vi "imageTrace.vi"() -> ()   [LabVIEW 2012]
uses:
  <vilib>/vision/NI_Vision_Development_Module.lvlib
panel:
  in  "Stop (F)":bool
  out "Image Out":T1(plugin-control)
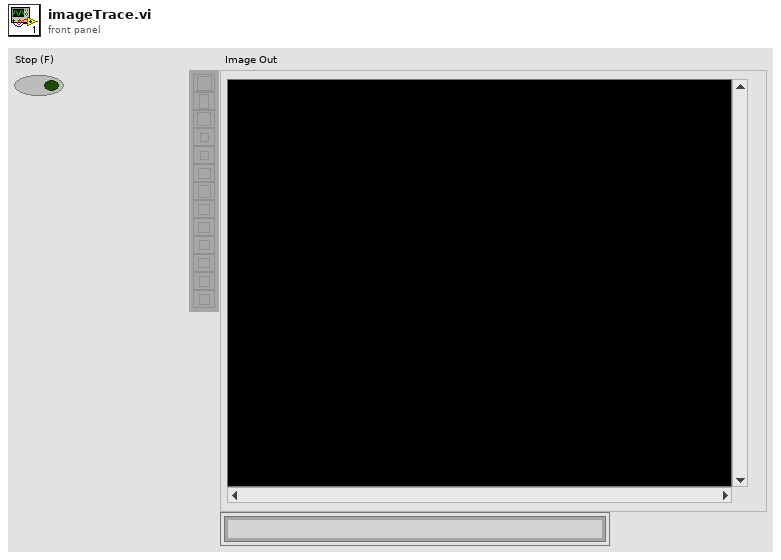
[diagram p1: front panel]
types:
  T1 = typedef "IMAQ Image.ctl" = refnum<image>
  T2 = typedef "Image Type" = u32
  T3 = cluster{"Position":cluster{"x":sgl, "y":sgl}, "Angle":sgl, "Scale":sgl, "Score":sgl, "Bounding Box":cluster{"x":sgl, "y":sgl}[]}[]
  T4 = cluster{"Matches (Pattern Matching 1)[0]":cluster{"Position":cluster{"x":sgl, "y":sgl}, "Angle":sgl, "Scale":sgl, "Score":sgl, "Bounding Box":cluster{"x":sgl, "y":sgl}[]}, "Matches (Pattern Matching 1)[1]":cluster{"Position":cluster{"x":sgl, "y":sgl}, "Angle":sgl, "Scale":sgl, "Score":sgl, "Bounding Box":cluster{"x":sgl, "y":sgl}[]}, "Matches (Pattern Matching 1)[2]":cluster{"Position":cluster{"x":sgl, "y":sgl}, "Angle":sgl, "Scale":sgl, "Score":sgl, "Bounding Box":cluster{"x":sgl, "y":sgl}[]}, "Matches (Pattern Matching 1)[3]":cluster{"Position":cluster{"x":sgl, "y":sgl}, "Angle":sgl, "Scale":sgl, "Score":sgl, "Bounding Box":cluster{"x":sgl, "y":sgl}[]}}
  T5 = cluster{"Bounding Box[0]":cluster{"x":sgl, "y":sgl}, "Bounding Box[1]":cluster{"x":sgl, "y":sgl}, "Bounding Box[2]":cluster{"x":sgl, "y":sgl}, "Bounding Box[3]":cluster{"x":sgl, "y":sgl}, "Bounding Box[4]":cluster{"x":sgl, "y":sgl}, "Bounding Box[5]":cluster{"x":sgl, "y":sgl}, "Bounding Box[6]":cluster{"x":sgl, "y":sgl}, "Bounding Box[7]":cluster{"x":sgl, "y":sgl}, "Bounding Box[8]":cluster{"x":sgl, "y":sgl}}
  T6 = cluster{"[0]":sgl, "[1]":sgl, "[2]":sgl, "[3]":sgl}
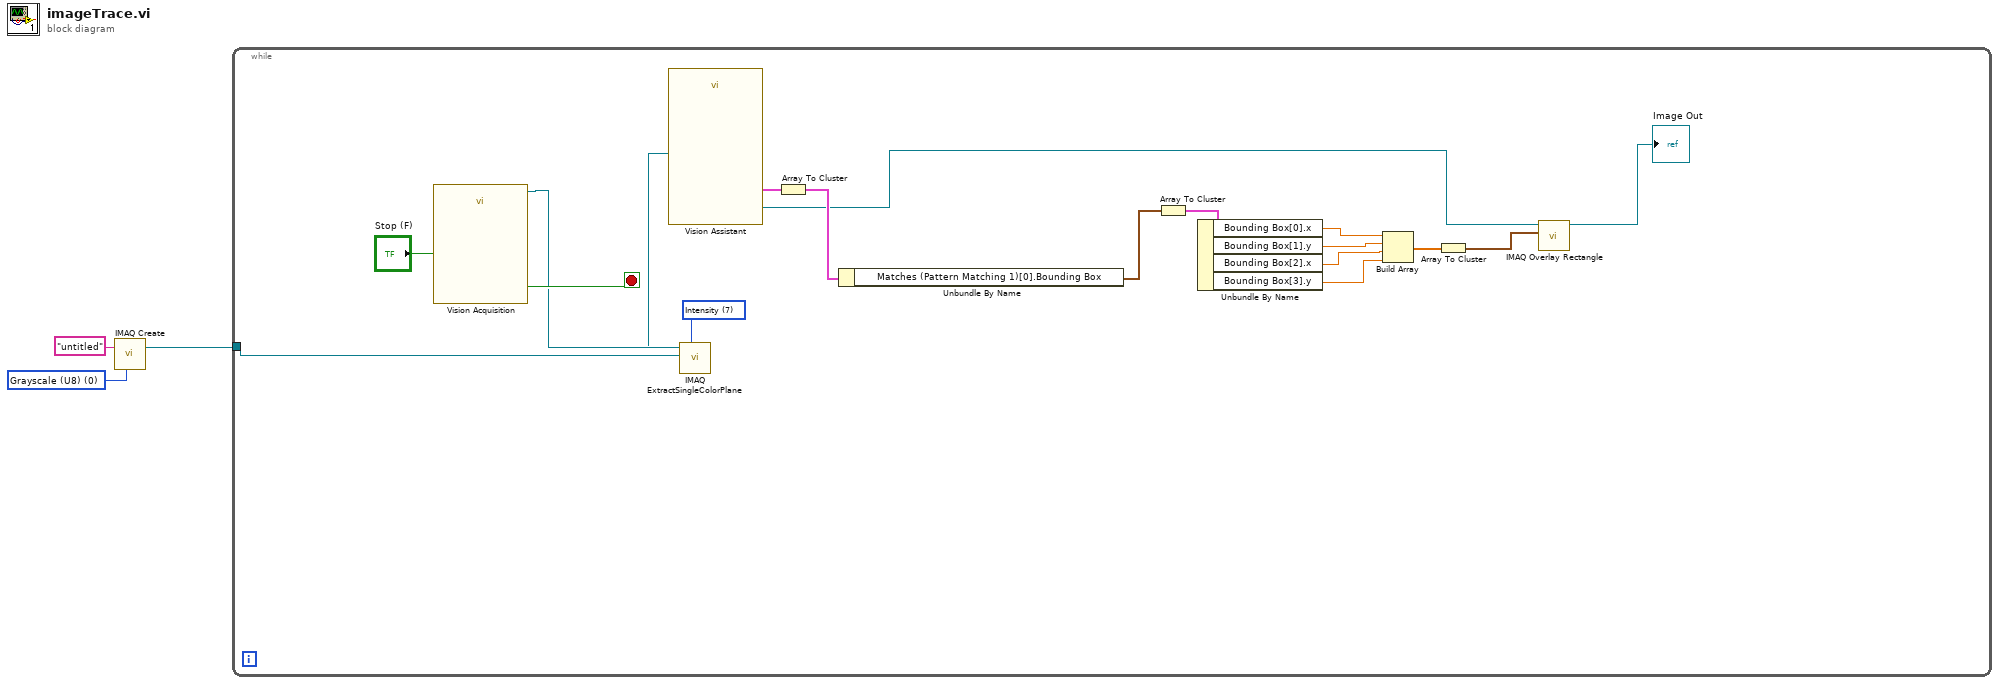
[diagram p0: block diagram]
diagram:
  w2 = T2 0 items=["Grayscale (U8)", "Grayscale (I16)", "Grayscale (SGL)", "Complex (CSG)", "RGB (U32)", "HSL (U32)", "RGB (U64)", "Grayscale (U16)"] ("Image Type")
  n1 = call "IMAQ Create"("Image Name"="untitled", "Image Type"=w2) -> ("New Image"=w1:T1)  [unwired: 3 in, 1 out]
  n2 = while {
    tunnel: w1 -> [w19]
    stop <- w20 stop-if-true
    w17 = 7 items=["Red", "Green", "Blue", "Hue", "Saturation", "Luminance", "Value", "Intensity"] ("Color Plane")
    n3 = call "Vision Acquisition"("Stop (F)"="Stop (F)") -> ("Image Out"=w18:T1, "Stopped"=w20:bool)  [unwired: 24 in, 1 out]
    n4 = call "IMAQ ExtractSingleColorPlane"("Color Plane"=w17, "Image Dst"=w19, "Image Src"=w18) -> ("Image Dst Out"=w16:T1)  [unwired: 7 in, 1 out]
    n5 = call "Vision Assistant"("Image In"=w16) -> ("Image Out"=w5:T1, "Matches (Pattern Matching 1)"=w15:T3)  [unwired: 24 in, 1 out]
    n6 = Array To Cluster(array=w15) -> (cluster=w14:T4)
    n7 = Unbundle By Name(w14) -> ("Matches (Pattern Matching 1)[0].Bounding Box"=w13:cluster{"x":sgl, "y":sgl}[])
    n8 = Array To Cluster(array=w13) -> (cluster=w12:T5)
    n9 = Unbundle By Name(w12) -> ("Bounding Box[0].x"=w11:sgl, "Bounding Box[1].y"=w10:sgl, "Bounding Box[2].x"=w9:sgl, "Bounding Box[3].y"=w8:sgl)
    n10 = Build Array(w11, w10, w9, w8) -> (w7:sgl[])
    n11 = Array To Cluster(array=w7) -> (cluster=w6:T6)
    n12 = call "IMAQ Overlay Rectangle"("Rectangle"=w6, "Image"=w5) -> ("Image Out"=→"Image Out":T1)  [unwired: 8 in, 1 out]
  }
